vi "Verify Checksum.vi"() -> ()   [LabVIEW 2010]
uses:
  Sensor Simulation Custom Device.lvlib
  Global.vi
  <vilib>/NI Veristand/Custom Device API/Custom Device API.lvlib
  <vilib>/NI VeriStand/Custom Device API/Get Item Property (String).vi
  <vilib>/NI VeriStand/Custom Device API/Get Item Property (Boolean).vi
  <vilib>/NI VeriStand/Custom Device API/Get Item Property (Dependent File).vi
  <userlib>/_FPGA Interface Advanced Tools/FPGA Bitfile Utility/FPGA Bitfile Utility.lvlib
  <vilib>/NI VeriStand/Custom Device API/Get Item Property (Dependent Node Pointer).vi
  <vilib>/NI Veristand/Custom Device API/Set Item Property (String).vi
  <vilib>/NI VeriStand/Custom Device API/Get Item Property (Variant).vi
  <vilib>/NI Veristand/Custom Device API/Set Item Property (Variant).vi
  TypeDefs/APUComp.ctl
  <vilib>/NI Veristand/Custom Device API/Custom Device Channel Type.ctl
  <vilib>/NI Veristand/Custom Device API/Custom Device Channel.ctl
  TypeDefs/NTeethComp.ctl
  <vilib>/NI Veristand/Custom Device API/Custom Device Item Ref.ctl
panel:
  in  "error in (no error)":errorcluster
  in  "Item Ref in":T1 format="%.0x"
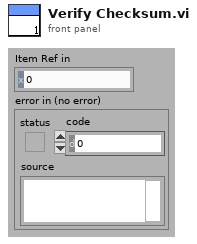
[diagram p1: front panel]
types:
  T1 = typedef "Custom Device API.lvlib/Custom Device Item Ref.ctl" = u64
  T2 = typedef "Sensor Simulation Custom Device.lvlib/NTeethComp.ctl" = cluster{"Name":string}
  T3 = typedef "Custom Device API.lvlib/Custom Device Channel.ctl" = cluster{"Type":T4, "Units":string, "Default Value":dbl, "Faultable":bool, "Scalable":bool}
  T4 = typedef "Custom Device API.lvlib/Custom Device Channel Type.ctl" = enum16{"Input", "Output"}
  T5 = typedef "Sensor Simulation Custom Device.lvlib/APUComp.ctl" = cluster{"Crank Angle":bool, "Cycle Angle":bool}
  T6 = typedef "FPGA Bitfile Utility.lvlib/Scalar Register Set.ctl" = cluster{"Boolean":T7[], "I8":T7[], "I16":T7[], "I32":T7[], "I64":T7[], "U8":T7[], "U16":T7[], "U32":T7[], "U64":T7[]}
  T7 = typedef "FPGA Bitfile Utility.lvlib/Scalar Register.ctl" = cluster{"Address":u32, "Name":string}
  T8 = typedef "FPGA Bitfile Utility.lvlib/FIFO Channel Set.ctl" = cluster{"Boolean":T9[], "I8":T9[], "I16":T9[], "I32":T9[], "I64":T9[], "U8":T9[], "U16":T9[], "U32":T9[], "U64":T9[]}
  T9 = typedef "FPGA Bitfile Utility.lvlib/FIFO Channel.ctl" = cluster{"Physical Channel":u32, "Name":string}
  T10 = cluster{string, "Indicator Scalars":T6, "Control Scalars":T6, "HostToTarget":T8}
  T11 = typedef "Sensor Simulation Custom Device.lvlib/EngineSimComps.ctl" = cluster{"LVDTs":T12[]}
  T12 = typedef "Sensor Simulation Custom Device.lvlib/LVDT.ctl" = cluster{"BitOffset":string, "ScaleFactor":string, "Number":i32}
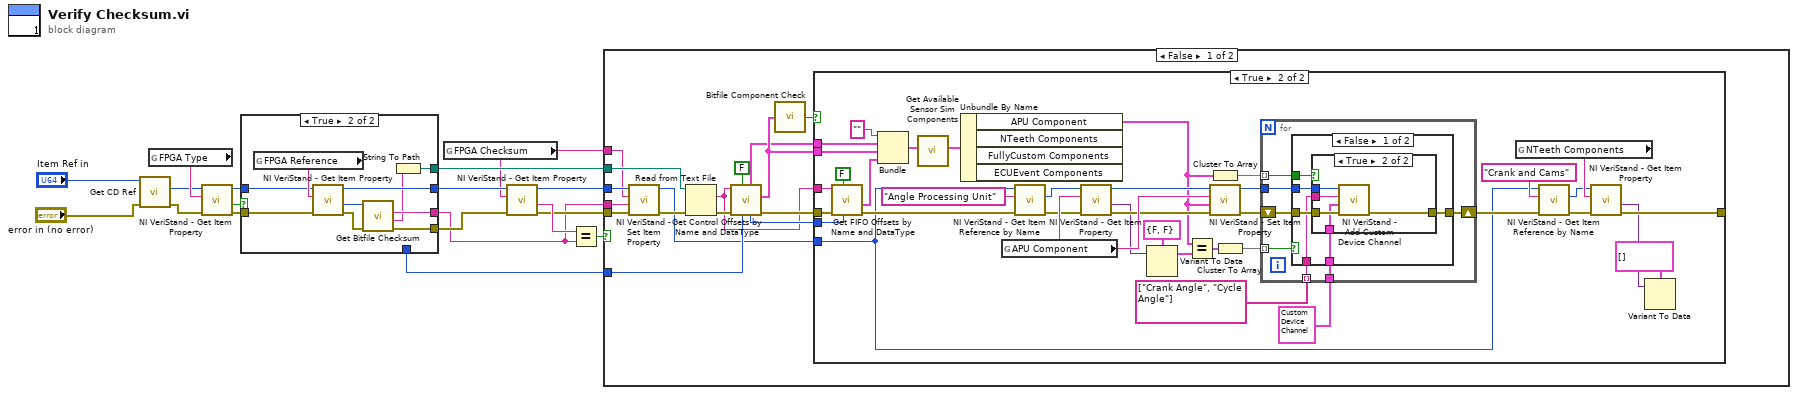
[diagram p0: block diagram]
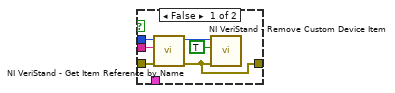
[diagram p3: hidden frame]
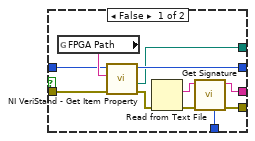
[diagram p6: hidden frame]
diagram:
  n1 = call "Get CD Ref.vi"("error in (no error)"="error in (no error)", "Item Ref in"="Item Ref in") -> ("error out"=w10:errorcluster, "CD Ref out"=w11:T1)  [unwired: 7 in, 1 out]
  n2 = global read "Global.vi" "FPGA Type"() -> (w15:string)
  n3 = call-poly <vilib>:"NI VeriStand - Get Item Property.vi"("error in (no error)"=w10, "Property Name"=w15, "Item Ref in"=w11) -> ("error out"=w12:errorcluster, "Value"=w14:bool, "Item Ref out"=w13:T1)  [unwired: 5 in, 1 out]
  n4 = case shown="True" w14 {
    tunnel: [w24 w39] -> w17
    tunnel: [w26 w35] -> w16
    tunnel: [w25 w34] -> w1
    tunnel: w13 -> [w28 w33]
    tunnel: w12 -> [w27 w32]
    tunnel: [w23 _] -> w6
    tunnel: [w22 w31] -> w4
    frame False {
      n5 = global read "Global.vi" "FPGA Path"() -> (w29:string)
      n6 = call-poly <vilib>:"NI VeriStand - Get Item Property.vi"("error in (no error)"=w27, "Property Name"=w29, "Item Ref in"=w28) -> ("error out"=w20:errorcluster, "Path"=w22:path, "Item Ref out"=w24:T1)  [unwired: 4 in, 2 out]
      n7 = Read from Text File(error in=w20) -> (text=w19:string, error out=w21:errorcluster)  [unwired: 3 in, 2 out]
      n8 = call <userlib>:"Get Signature.vi"("error in (no error)"=w21, "bitfile xml in"=w19) -> ("error out"=w26:errorcluster, "Bitfile Signature"=w25:string, "offset past EndTag"=w23:i32)  [unwired: 7 in]
    }
    frame True {
      n9 = global read "Global.vi" "FPGA Reference"() -> (w38:string)
      n10 = call-poly <vilib>:"NI VeriStand - Get Item Property.vi"("error in (no error)"=w32, "Property Name"=w38, "Item Ref in"=w33) -> ("error out"=w36:errorcluster, "Dependent Node Ref"=w37:T1, "Item Ref out"=w39:T1)  [unwired: 5 in, 1 out]
      n11 = call "Get Bitfile Checksum.vi"("error in (no error)"=w36, "ID in"=w37) -> ("error out"=w35:errorcluster, "Path"=w30:string, "MD5"=w34:string)  [unwired: 6 in, 1 out]
      n12 = String To Path(string=w30) -> (path=w31:path)
    }
  }
  n13 = global read "Global.vi" "FPGA Checksum"() -> (w2:string)
  n14 = call-poly <vilib>:"NI VeriStand - Get Item Property.vi"("error in (no error)"=w16, "Property Name"=w2, "Item Ref in"=w17) -> ("error out"=w7:errorcluster, "Value"=w8:string, "Item Ref out"=w3:T1)  [unwired: 5 in, 1 out]
  n15 = Equal?(x=w8, y=w1) -> (x = y?=w5:bool)
  n16 = case shown="False" w5 {
    tunnel: w7 -> [w46 _]
    tunnel: w6 -> [w49 _]
    tunnel: w4 -> [w47 _]
    tunnel: w3 -> [w44 _]
    tunnel: w2 -> [w43 _]
    tunnel: w1 -> [w42 _]
    frame False {
      n17 = call-poly <vilib>:"NI VeriStand - Set Item Property.vi"("error in (no error)"=w46, "Value"=w42, "Property Name"=w43, "Item Ref in"=w44) -> ("error out"=w45:errorcluster, "Item Ref out"=w41:T1)  [unwired: 5 in, 1 out]
      n18 = Read from Text File(file (use dialog)=w47, error in=w45) -> (text=w40:string, error out=w48:errorcluster)  [unwired: 2 in, 2 out]
      n19 = call <userlib>:"Get Control Offsets by Name and DataType.vi"("offset"=w49, "User Specified?"=FALSE, "error in"=w48, "bitfile xml in"=w40) -> ("error out"=w54:errorcluster, "Control Scalars"=w52:T6, "offset past EndTag"=w50:i32, "Indicator Scalars"=w51:T6)  [unwired: 2 in, 2 out]
      n20 = call "Bitfile Component Check.vi"("Control Scalars"=w52) -> ("Valid?"=w53:bool)
      n21 = case shown="True" w53 {
        tunnel: w54 -> [w56 w93]
        tunnel: w52 -> [_ w91]
        tunnel: w51 -> [_ w90]
        tunnel: [w56 w67] -> _
        tunnel: w50 -> [_ w88]
        tunnel: w41 -> [_ w62]
        tunnel: w40 -> [_ w57]
        frame False {
        }
        frame True {
          n22 = call <userlib>:"Get FIFO Offsets by Name and DataType.vi"("offset"=w88, "User Specified?"=FALSE, "error in"=w93, "bitfile xml in"=w57) -> ("error out"=w82:errorcluster, "HostToTarget"=w92:T8)  [unwired: 3 in, 3 out]
          n23 = Bundle("", "Indicator Scalars"=w90, "Control Scalars"=w91, "HostToTarget"=w92) -> (w86:T10)  [unwired: 1 in]
          n24 = call "Get Available Sensor Sim Components.vi"("Register Info"=w86) -> ("Sensor Sim Components"=w85:T11)  [unwired: 9 in, 1 out]
          n25 = Unbundle By Name(w85) -> ("APU Component"=w71:T5)  [unwired: 3 out]
          n26 = global read "Global.vi" "APU Component"() -> (w84:string)
          n27 = call <vilib>:"NI VeriStand - Get Item Reference by Name.vi"("error in (no error)"=w82, "Item Name"="Angle Processing Unit", "Parent Ref in"=w62) -> ("error out"=w80:errorcluster, "Item Ref"=w66:T1)  [unwired: 5 in, 2 out]
          n28 = call-poly <vilib>:"NI VeriStand - Get Item Property.vi"("error in (no error)"=w80, "Property Name"=w84, "Item Ref in"=w66) -> ("error out"=w83:errorcluster, "Value"=w78:variant, "Item Ref out"=w79:T1)  [unwired: 5 in, 1 out]
          n29 = Variant To Data(Variant=w78, type=T5 {"Crank Angle"=FALSE, "Cycle Angle"=FALSE} ("APU Component")) -> (data=w76:T5)  [unwired: 1 in, 1 out]
          n30 = Equal?(x=w71, y=w76) -> (x = y?=w75:T5)
          n31 = Cluster To Array(cluster=w71) -> (array=w70:bool[])
          n32 = call-poly <vilib>:"NI VeriStand - Set Item Property.vi"("error in (no error)"=w83, "Value"=w71, "Property Name"=w84, "Item Ref in"=w79) -> ("error out"=w73:errorcluster, "Item Ref out"=w74:T1)  [unwired: 5 in, 1 out]
          n33 = Cluster To Array(cluster=w75) -> (array=w72:bool[])
          n34 = for {
            tunnel: w74 -> [w99]
            shift-right: [w94] -> w63
            shift-left: w73 -> [w98]
            tunnel: w72 -> [w100] mode=indexing
            tunnel: w70 -> [w97] mode=indexing
            tunnel: string[] ["Crank Angle", "Cycle Angle"] -> [w96] mode=indexing
            tunnel: T3 {"Type"=enum."Output", "Units"="Degrees", "Default Value"=0.0, "Faultable"=FALSE, "Scalable"=FALSE} ("Channel") -> [w95]
            n35 = case shown="False" w100 {
              tunnel: w99 -> [w105 _]
              tunnel: w98 -> [w104 w118]
              tunnel: w97 -> [w106 _]
              tunnel: w96 -> [w103 _]
              tunnel: w95 -> [w102 _]
              tunnel: [w101 w118] -> w94
              frame False {
                n36 = case shown="True" w106 {
                  tunnel: w105 -> [w112 w117]
                  tunnel: w104 -> [w111 w115]
                  tunnel: w103 -> [w110 w116]
                  tunnel: w102 -> [_ w114]
                  tunnel: [w107 w113] -> w101
                  frame False {
                    n37 = call <vilib>:"NI VeriStand - Get Item Reference by Name.vi"("error in (no error)"=w111, "Item Name"=w110, "Parent Ref in"=w112) -> ("error out"=w107:errorcluster, "Parent Ref out"=w109:T1)  [unwired: 5 in, 2 out]
                    n38 = call <vilib>:"NI VeriStand - Remove Custom Device Item.vi"("error in (no error)"=w107, "Force Delete (F)"=TRUE, "Item Ref in"=w109) -> ()  [unwired: 7 in, 2 out]
                  }
                  frame True {
                    n39 = call <vilib>:"NI VeriStand - Add Custom Device Channel.vi"("error in (no error)"=w115, "Channel"=w114, "Channel Name"=w116, "Parent Ref in"=w117) -> ("error out"=w113:errorcluster)  [unwired: 4 in, 3 out]
                  }
                }
              }
              frame True {
              }
            }
          }
          n40 = global read "Global.vi" "NTeeth Components"() -> (w65:string)
          n41 = call <vilib>:"NI VeriStand - Get Item Reference by Name.vi"("error in (no error)"=w63, "Item Name"="Crank and Cams", "Parent Ref in"=w62) -> ("error out"=w60:errorcluster, "Item Ref"=w61:T1)  [unwired: 5 in, 2 out]
          n42 = call-poly <vilib>:"NI VeriStand - Get Item Property.vi"("error in (no error)"=w60, "Property Name"=w65, "Item Ref in"=w61) -> ("error out"=w67:errorcluster, "Value"=w59:variant)  [unwired: 5 in, 2 out]
          n43 = Variant To Data(Variant=w59, type=T2[] [] ("NTeeth Components")) -> ()  [unwired: 1 in, 2 out]
        }
      }
    }
    frame True {
    }
  }
